vi "Try Match Response.vi"(8 "error in":errorcluster, 10 "ICAN CC Frame":refnum<class "ICAN CC Frame.lvclass">, 11 "Expedited Download Transfer in":refnum<class "Download Expedited Transfer.lvclass">) -> (0 "error out":errorcluster, 2 "Match":bool, 3 "Expedited Download Transfer out":refnum<class "SDO Transfer.lvclass">)   [LabVIEW 2020, in "CANopen.lvlib" / "SDO Manager.lvlib" / "Download Expedited Transfer.lvclass"]
uses:
  Download Expedited Transfer.lvclass
  D:/git/CANopen-LabVIEW/source/SDO Manager/SDO Manager/SDO Transfer/SDO Transfer.lvclass
  SDO Transfer/SDO Transfer.lvclass
  HAL/Source/Interfaces/ICAN CC Frame/ICAN CC Frame.lvclass
  D:/git/HAL/Source/Interfaces/IMessage/IMessage.lvclass
  SDO Transfer/SDO Transfer.lvclass/SDO Transfer.ctl
  SDO Transfer/SDO abort code.ctl
  CANopen Message/CANopen Message.lvclass
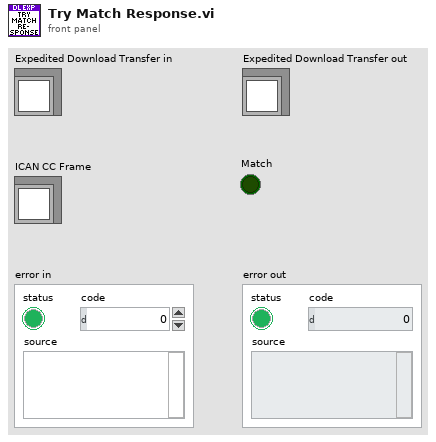
[diagram p1: front panel]
types:
  T1 = typedef "CANopen.lvlib/SDO Manager.lvlib/SDO Transfer.lvclass/SDO abort code.ctl" = u32
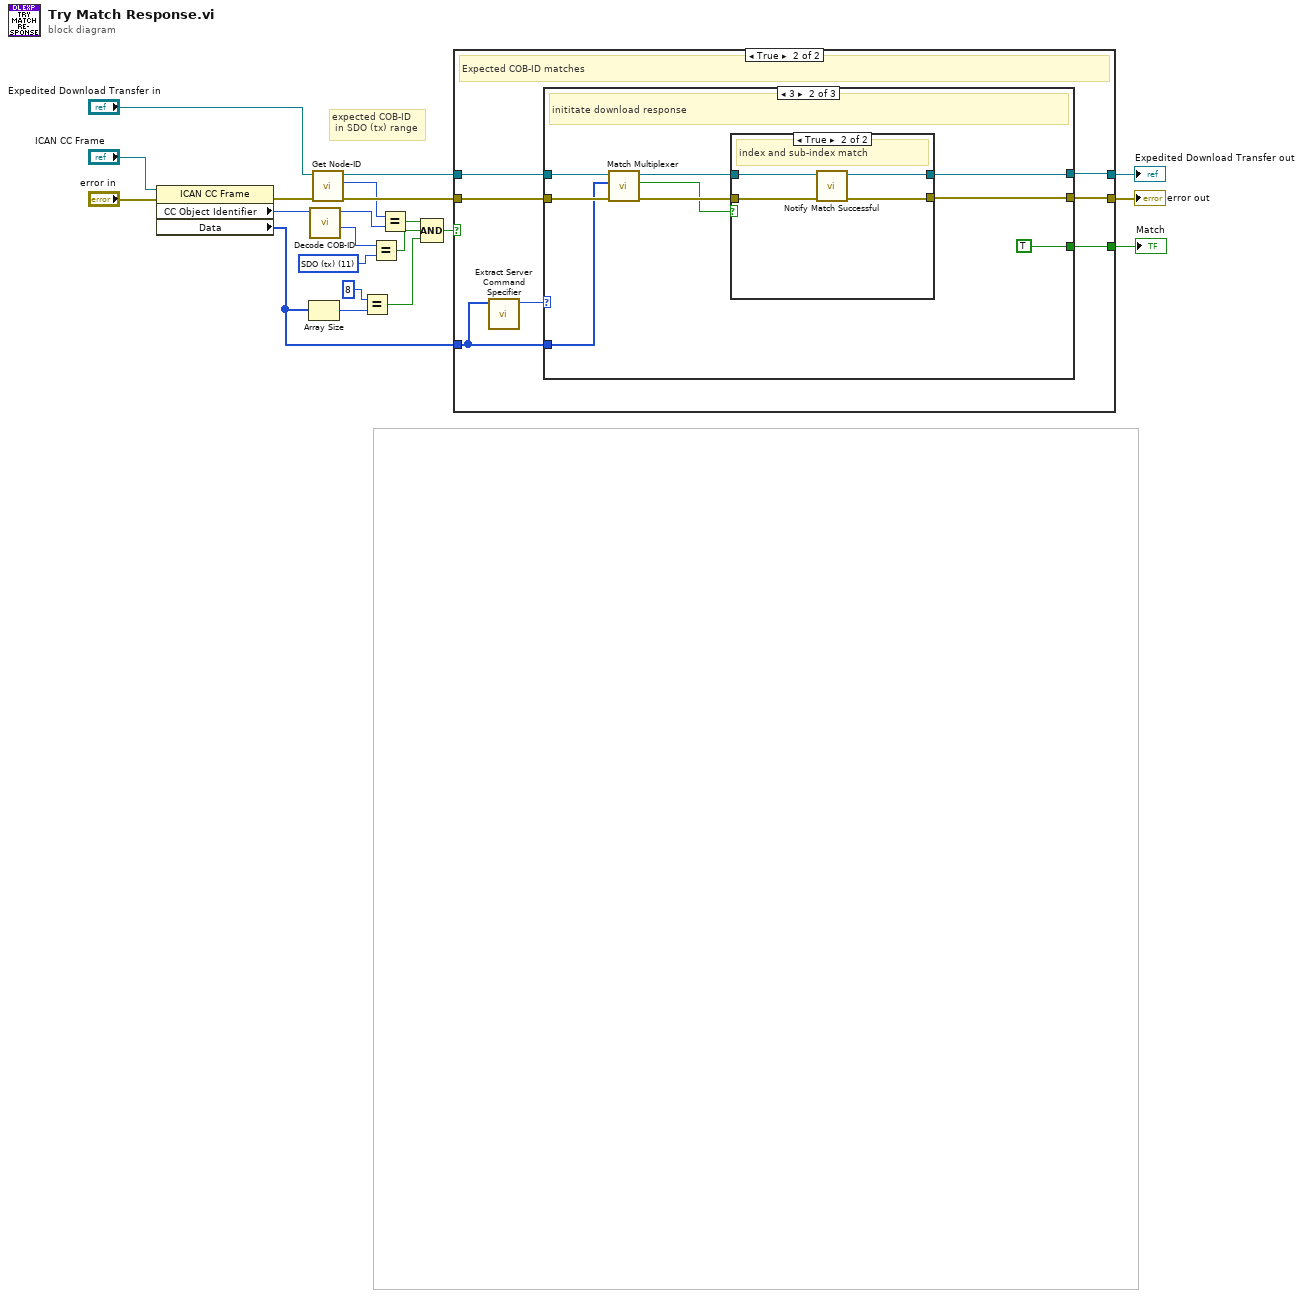
[diagram p0: block diagram]
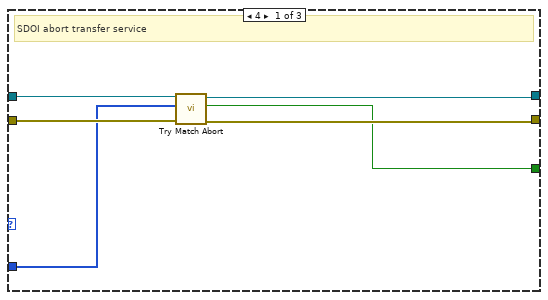
[diagram p3: hidden frame]
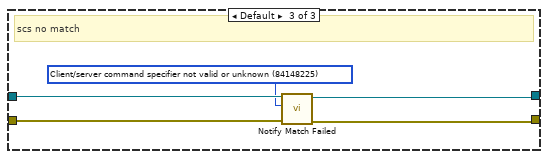
[diagram p5: hidden frame]
diagram:
  w7 = u8 11 items=["NMT"=0, "EMCY/SYNC"=1, "TIME"=2, "PDO1 (tx)"=3, "PDO1 (rx)"=4, "PDO2 (tx)"=5, "PDO2 (rx)"=6, "PDO3 (tx)"=7, "PDO3 (rx)"=8, "PDO4 (tx)"=9, "PDO4 (rx)"=10, "SDO (tx)"=11, "SDO (rx)"=12, "NMT error control"=14] ("Function Code")
  # "expected COB-ID\n in SDO (tx) range"
  n1 = property class="ICAN CC Frame"(reference="ICAN CC Frame", error in="error in") -> (error out=w19:errorcluster, "CC Object Identifier"=w11:u32, "Data"=w2:u8[])  [unwired: 1 out]
  n2 = Array Size(array=w2) -> (size(s)=w4:i32)
  n3 = call "Decode COB-ID.vi"("COD-ID"=w11) -> ("Function Code"=w6:u8, "Node-ID"=w10:u8)  [unwired: 9 in]
  n4 = call "Get Node-ID.vi"("error in"=w19, "SDO Transfer in"="Expedited Download Transfer in") -> ("error out"=w16:errorcluster, "Node-ID"=w9:u8, "SDO Transfer out"=w17:refnum<class "Download Expedited Transfer.lvclass">)  [unwired: 7 in]
  n5 = Equal?(x=8, y=w4) -> (x = y?=w1:bool)
  n6 = Equal?(x=w6, y=w7) -> (x = y?=w5:bool)
  n7 = Equal?(x=w9, y=w10) -> (x = y?=w15:bool)
  n8 = Compound Arithmetic op=AND(w15, w5, w1) -> (w8:bool)
  n9 = case shown="True" w8 {
    tunnel: w17 -> [w23 w30]
    tunnel: w16 -> [w22 w29]
    tunnel: [w23 w27] -> w14
    tunnel: [w22 w28] -> w13
    tunnel: w2 -> [_ w25]
    tunnel: [_ w26] -> w12
    frame False {
    }
    frame True {
      # "Expected COB-ID matches"
      n10 = call "Extract Server Command Specifier.vi"("Data"=w25) -> ("Server Command Specifier"=w24:u8)  [unwired: 10 in]
      n11 = case shown="3" w24 {
        tunnel: w30 -> [w35 w40 w55]
        tunnel: w29 -> [w36 w45 w56]
        tunnel: [w32 w43 w54] -> w27
        tunnel: [w33 w44 w53] -> w28
        tunnel: [w31 TRUE _] -> w26
        tunnel: w25 -> [w34 w38 _]
        frame 4 {
          # "SDOI abort transfer service"
          n12 = call "Try Match Abort.vi"("error in"=w36, "Frame Data"=w34, "SDO Transfer in"=w35) -> ("error out"=w33:errorcluster, "Match"=w31:bool, "SDO Transfer out"=w32:refnum<class "Download Expedited Transfer.lvclass">)  [unwired: 6 in]
        }
        frame 3 {
          # "inititate download response"
          n13 = call "Match Multiplexer.vi"("error in"=w45, "Frame Data"=w38, "SDO Transfer in"=w40) -> ("error out"=w41:errorcluster, "Match"=w37:bool, "SDO Transfer out"=w39:refnum<class "Download Expedited Transfer.lvclass">)  [unwired: 6 in]
          n14 = case shown="True" w37 {
            tunnel: w41 -> [w47 w51]
            tunnel: [w47 w50] -> w44
            tunnel: w39 -> [w46 w49]
            tunnel: [w46 w48] -> w43
            frame False {
              # "index or sub-index no match"
            }
            frame True {
              # "index and sub-index match"
              n15 = call "Notify Match Successful.vi"("error in"=w51, "SDO Transfer in"=w49) -> ("error out"=w50:errorcluster, "SDO Transfer out"=w48:refnum<class "Download Expedited Transfer.lvclass">)  [unwired: 8 in]
            }
          }
        }
        frame Default {
          w52 = T1 84148225 items=["Toggle bit not allowed"=84082688, "SDO protocol timed out"=84148224, "Client/server command specifier not valid or unknown"=84148225, "Invalid block size (block mode only)"=84148226, "Invalid sequence number (block mode only)"=84148227, "CRC error (block mode only)"=84148228, "Out of memory"=84148229, "Attempt to read a write only object"=100728833, "Attempt to write a read only object"=100728834, "Object does not exist in the object dictionary"=100794368, "Object cannot be mapped to the PDO"=100925505, "The number and length of the objects to be mapped would exceed PDO length"=100925506, "General parameter incompatibility reason"=100925507, "General internal incompatibility in the device"=100925511, "Access failed due to an hardware error"=101056512, "Data type does not match, length of service parameter does not match"=101122064, "Data type does not match, length of service parameter too high"=101122066, "Data type does not match, length of service parameter too low"=101122067, "Sub-index does not exist"=101253137, "Invalid value for parameter (download only)"=101253168, "Value of parameter written too high (download only)"=101253169, "Value of parameter written too low (download only)"=101253170, "Maximum value is less than minimum value"=101253174, "Resource not available: SDO connection"=101318691, "General error"=134217728, "Data cannot be transferred or stored to the application"=134217760, "Data cannot be transferred or stored to the application because of local control"=134217761, "Data cannot be transferred or stored to the application because of the present device stable"=134217762, "Object dictionary dynamic generation fails or no object dictionary is present (e.g. object dictionary is generated from file and generation fails because of an file error)"=134217763, "No data available"=134217764] ("SDO abort code")
          # "scs no match"
          n16 = call "Notify Match Failed.vi"("error in"=w56, "SDO abort code"=w52, "SDO Transfer in"=w55) -> ("error out"=w53:errorcluster, "SDO Transfer out"=w54:refnum<class "Download Expedited Transfer.lvclass">)  [unwired: 7 in]
        }
      }
    }
  }
  "Expedited Download Transfer out" <- w14
  "error out" <- w13
  "Match" <- w12
